vi "Execute.Initialize.vi"(8 "error in (no error)":errorcluster, 11 "Cluster":T1) -> (0 "error out":errorcluster)   [LabVIEW 2015, in "Station.Execution.lvlib"]
uses:
  Station.Execution.lvlib
  Types/Main.StateVariables.ctl
  Types/Execute.UserEventRefs.ctl
  <vilib>/NI Veristand/Execution/Workspace/SystemStateRegEventRef.ctl
  <vilib>/NI Veristand/Execution/Workspace/Target State Info.ctl
  <vilib>/NI Veristand/Execution/Workspace/Target State.ctl
  <vilib>/NI Veristand/Execution/Workspace/SystemStateEventRef.ctl
  <vilib>/NI Veristand/Execution/Workspace/WorkspaceAPI.ctl
  NationalInstruments.VeriStand.ClientAPI
  Types/UI.Tables.ctl
  Types/UI.Object.ctl
  <vilib>/NI Veristand/Execution/Workspace/NI_VS Workspace ExecutionAPI.lvlib
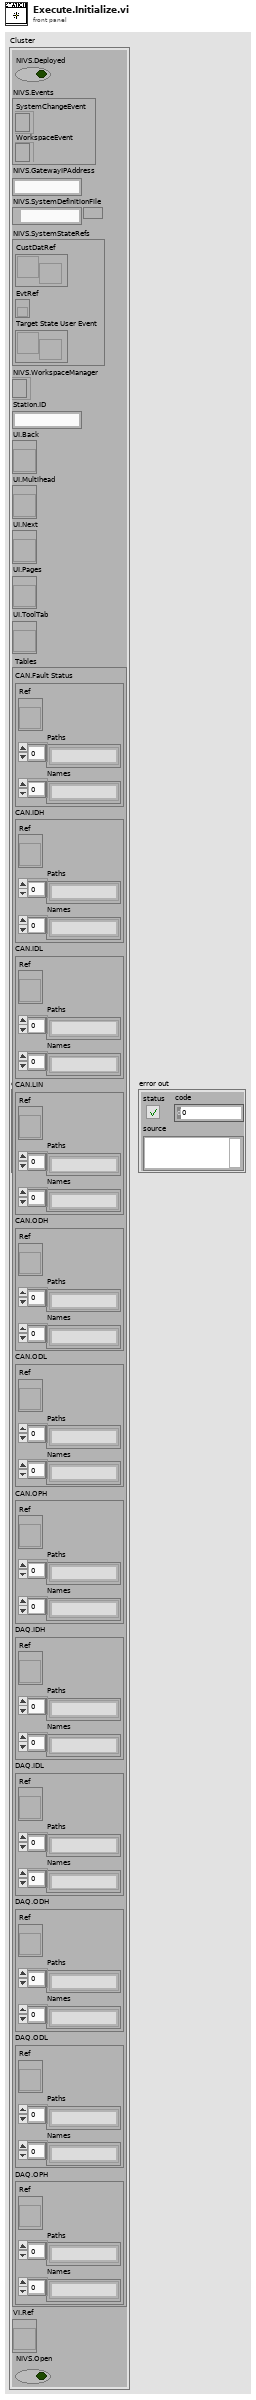
[diagram p1: front panel]
types:
  T1 = typedef "Station.Execution.lvlib/Main.StateVariables.ctl" = cluster{"NIVS.Deployed":bool, "NIVS.Events":T2, "NIVS.GatewayIPAddress":string, "NIVS.SystemDefinitionFile":path, "NIVS.SystemStateRefs":T4, "NIVS.WorkspaceManager":T5, "Station.ID":string, "UI.Back":refnum<vi>, "UI.Multihead":refnum<vi>, "UI.Next":refnum<vi>, "UI.Pages":refnum<vi>, "UI.ToolTab":refnum<vi>, "Tables":T6, "VI.Ref":refnum<vi>, "NIVS.Open":bool}
  T2 = typedef "Station.Execution.lvlib/Execute.UserEventRefs.ctl" = cluster{"SystemChangeEvent":T3, "WorkspaceEvent":refnum<event-registration>}
  T3 = typedef "NI_VS Workspace ExecutionAPI.lvlib/SystemStateRegEventRef.ctl" = refnum<event-registration>
  T4 = typedef "NI_VS Workspace ExecutionAPI.lvlib/SystemStateEventRef.ctl" = cluster{"CustDatRef":refnum<user-event>, "EvtRef":refnum<k27>, "Target State User Event":refnum<user-event>}
  T5 = typedef "NI_VS Workspace ExecutionAPI.lvlib/WorkspaceAPI.ctl" = refnum<k24>
  T6 = typedef "Station.Execution.lvlib/UI.Tables.ctl" = cluster{"CAN.Fault Status":T7, "CAN.IDH":T7, "CAN.IDL":T7, "CAN.LIN":T7, "CAN.ODH":T7, "CAN.ODL":T7, "CAN.OPH":T7, "DAQ.IDH":T7, "DAQ.IDL":T7, "DAQ.ODH":T7, "DAQ.ODL":T7, "DAQ.OPH":T7}
  T7 = typedef "Station.Execution.lvlib/UI.Object.ctl" = cluster{"Ref":refnum<vi>, "Paths":string[], "Names":string[]}
  T8 = enum8{"Enabled", "Disabled", "Disabled and Grayed Out"}
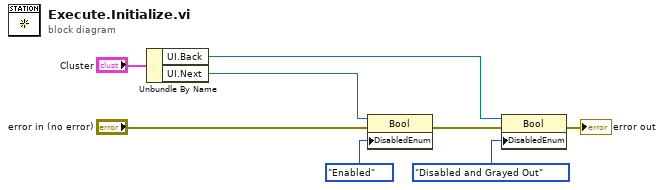
[diagram p0: block diagram]
diagram:
  n1 = Unbundle By Name("Cluster") -> ("UI.Back"=w5:refnum<vi>, "UI.Next"=w6:refnum<vi>)
  n2 = property class="Bool"(reference=w6, error in="error in (no error)", "DisabledEnum"=T8."Enabled" ("Disabled")) -> (error out=w7:errorcluster)  [unwired: 1 out]
  n3 = property class="Bool"(reference=w5, error in=w7, "DisabledEnum"=T8."Disabled and Grayed Out" ("Disabled")) -> (error out=→"error out":errorcluster)  [unwired: 1 out]
